vi "_TangoAttributeDataReadyEventGroupKill.vi"(1 "error in":errorcluster, 2 "attribute data ready event ref":T1) -> (0 "error out":errorcluster)   [LabVIEW 2014, in "tango.lvlib"]
uses:
  tango.lvlib
  Common VIs/Typedefs/_AttributeDataReadyEventRef.ctl
  tango_binding.so
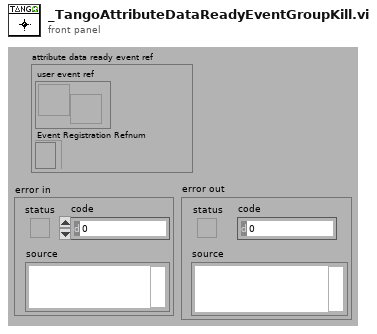
[diagram p1: front panel]
types:
  T1 = typedef "tango.lvlib/_AttributeDataReadyEventRef.ctl" = cluster{"user event ref":refnum<user-event>, "user event reg refnum":refnum<event-registration>}
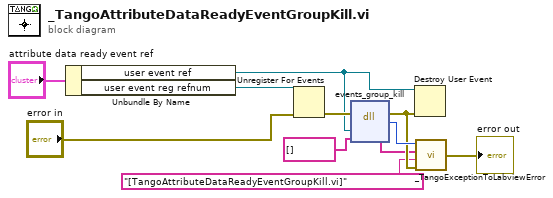
[diagram p0: block diagram]
diagram:
  n1 = Unbundle By Name("attribute data ready event ref") -> ("user event ref"=w2:refnum<user-event>, "user event reg refnum"=w3:refnum<event-registration>)
  n2 = Unregister For Events(event registration refnum=w3, error in="error in") -> (error out=w11:errorcluster)
  n3 = dll-call lib="tango_binding.*" fn="events_group_kill"(error in=w11, "event refnum"=w2, "error_stack"=string[] []) -> (error out=w7:errorcluster, "return type"=w8:i32, "error_stack"=w6:string[])  [unwired: 3 in, 1 out]
  n4 = Destroy User Event(user event=w2, error in=w7) -> ()  [unwired: 1 out]
  n5 = call "_TangoExceptionToLabviewError.vi"("error in"=w7, "location"="[TangoAttributeDataReadyEventGroupKill.vi]", "error stack"=w6, "error code"=w8) -> ("error out"=→"error out":errorcluster)
